vi "Class Test Harness.vi"() -> ()   [LabVIEW 2017]
uses:
  Simple Actor/Simple Actor/Simple Actor.lvclass
  Simple Actor/Simple Actor/Simple Actor.lvclass/Simple Actor.ctl
panel:
  out "Time":dbl
  in  "Update":bool
  in  "Process Stop Button":bool
  in  "Zero Button":bool
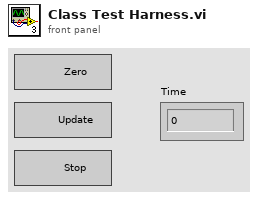
[diagram p1: front panel]
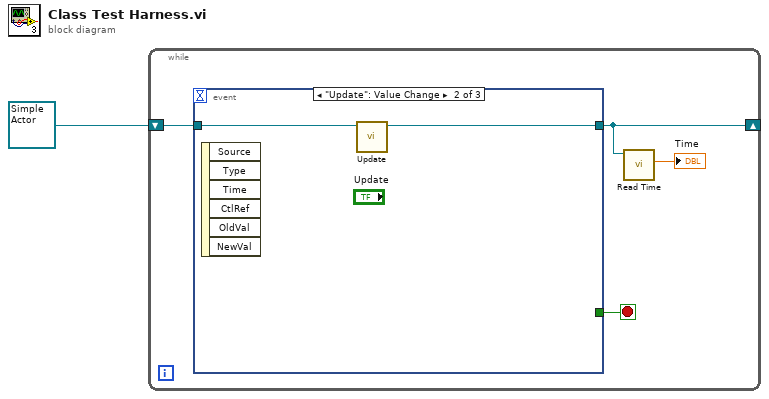
[diagram p0: block diagram]
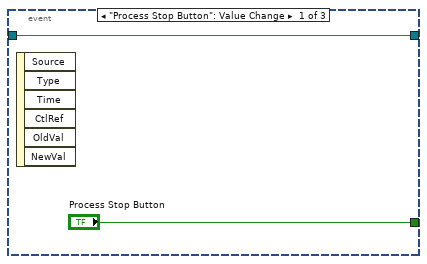
[diagram p2: hidden frame]
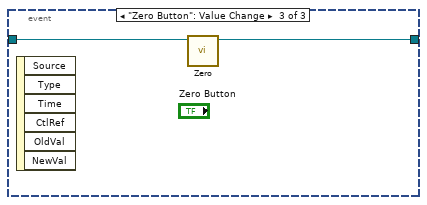
[diagram p3: hidden frame]
diagram:
  n1 = while {
    shift-right: [w3] -> _
    shift-left: refnum<class "Simple Actor.lvclass"> refnum ("Simple Actor.lvlib:Simple Actor.lvclass") -> [w4]
    stop <- w5 stop-if-true
    n2 = event shown="[1] \"Update\": Value Change" {
      selector: _ -> [_ _ _]
      dyn-events: _ -> [_ _ _]
      timeout: _ -> [_ _ _]
      tunnel: ["Process Stop Button" _ _] -> w5
      tunnel: [w6 w8 w10] -> w3
      tunnel: w4 -> [w6 w9 w11]
      event "Process Stop Button": Value Change {
        n3 = event-data() -> ()  [unwired: 1 in, 6 out]
      }
      event "Update": Value Change {
        n4 = event-data() -> ()  [unwired: 1 in, 6 out]
        n5 = call "Update.vi"("Simple Actor in"=w9) -> ("Simple Actor out"=w8:refnum<class "Simple Actor.lvclass">)  [unwired: 10 in]
      }
      event "Zero Button": Value Change {
        n6 = event-data() -> ()  [unwired: 1 in, 6 out]
        n7 = call "Zero.vi"("Simple Actor in"=w11) -> ("Simple Actor out"=w10:refnum<class "Simple Actor.lvclass">)  [unwired: 9 in, 1 out]
      }
    }
    n8 = call "Read Time.vi"("Simple Actor in"=w3) -> ("Time"=→"Time":dbl)  [unwired: 10 in]
  }
